vi "Cut.vi"(8 "error in (no error)":errorcluster, 11 "ChicagoStyleCheesePizza in":refnum<class "ChicagoStyleCheesePizza.lvclass">) -> (0 "error out":errorcluster, 3 "ChicagoStyleCheesePizza out":refnum<class "ChicagoStyleCheesePizza.lvclass">)   [LabVIEW 2020, in "FactoryMethod.lvlib" / "PizzaFactoryMethod.lvlib" / "ChicagoStyleCheesePizza.lvclass"]
uses:
  ChicagoStyleCheesePizza.lvclass
  Support/Class/ConsoleOutput.lvclass
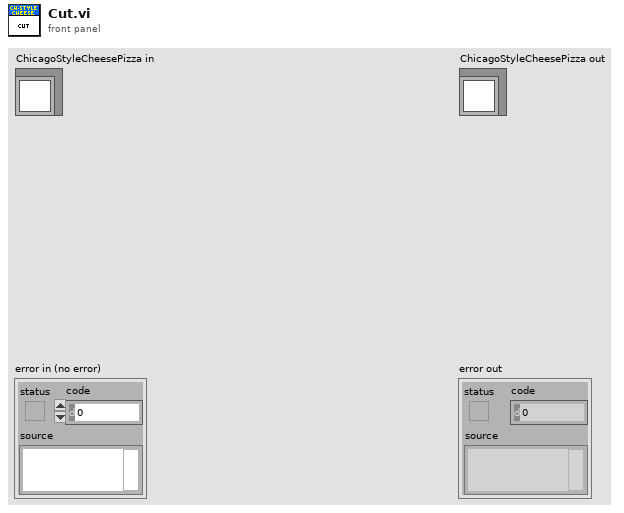
[diagram p1: front panel]
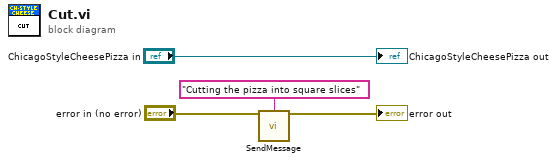
[diagram p0: block diagram]
diagram:
  n1 = call "SendMessage.vi"("Message"="Cutting the pizza into square slices", "error in (no error)"="error in (no error)") -> ("error out"=→"error out":errorcluster)  [unwired: 13 in]
  "ChicagoStyleCheesePizza out" <- "ChicagoStyleCheesePizza in"
